vi "Start.vi"(8 "error in (no error)":errorcluster, 11 "MQTT_Base in":refnum<class "MQTT_Base.lvclass">) -> (0 "error out":errorcluster, 1 "timed out?":bool, 3 "MQTT_Base out":refnum<class "MQTT_Base.lvclass">)   [LabVIEW 2013, in "MQTT Base.lvlib" / "MQTT_Base.lvclass"]
uses:
  MQTT_Base.lvclass
  MQTT_Base.lvclass/MQTT_Base.ctl
  Launch Async Process.vi
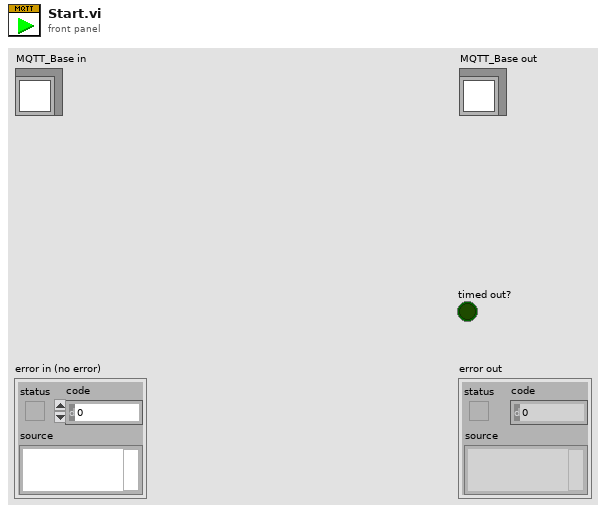
[diagram p1: front panel]
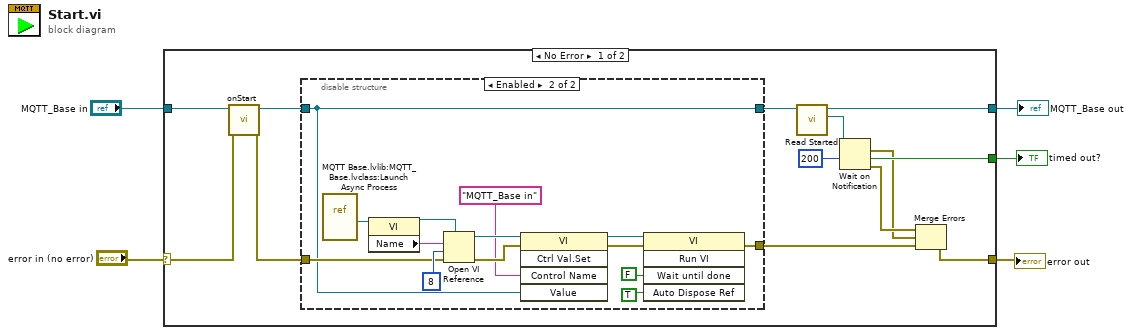
[diagram p0: block diagram]
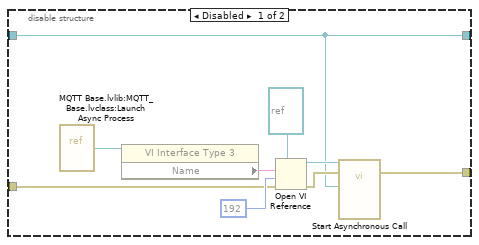
[diagram p2: hidden frame]
diagram:
  n1 = case shown="No Error" "error in (no error)" {
    selector: "error in (no error)" -> [w12 w43]
    tunnel: [w14 w43] -> w3
    tunnel: [w9 w42] -> w2
    tunnel: "MQTT_Base in" -> [w13 w42]
    tunnel: [w16 _] -> w1
    frame No Error {
      n2 = call-dynamic "onStart.vi"("error in (no error)"=w12, "MQTT_Base in"=w13) -> ("error out"=w11:errorcluster, "MQTT_Base out"=w8:refnum<class "MQTT_Base.lvclass">)  [unwired: 8 in]
      n3 = disable-structure shown="Enabled" {
        disable-tunnel: w11 -> [w23 w37]
        disable-tunnel: w8 -> [w21 w28]
        disable-tunnel: [w22 w32] -> w7
        disable-tunnel: [w21 w28] -> w6
        frame Disabled {
          n4 = vi-ref "MQTT Base.lvlib:MQTT_Base.lvclass:Launch Async Process.vi"() -> (w19:refnum<vi>)
          n5 = property class="VI Interface Type 3"(reference=w19) -> ("Name"=w27:string)  [unwired: 1 in, 2 out]
          n6 = Open VI Reference(type specifier VI Refnum (for type only)=refnum<vi> refnum ("reference out"), vi path=w27, options=192, error in (no error)=w23) -> (vi reference=w26:refnum<vi>, error out=w25:errorcluster)  [unwired: 2 in]
          n7 = call-by-ref "Start Asynchronous Call"(reference=w26, error in=w25, "MQTT_Base in"=w21) -> (error out=w22:errorcluster)  [unwired: 11 in, 1 out]
        }
        frame Enabled {
          n8 = vi-ref "MQTT Base.lvlib:MQTT_Base.lvclass:Launch Async Process.vi"() -> (w41:refnum<vi>)
          n9 = property class="VI"(reference=w41) -> (reference out=w39:refnum<vi>, "Name"=w40:string)  [unwired: 1 in, 1 out]
          n10 = Open VI Reference(type specifier VI Refnum (for type only)=w39, vi path=w40, options=8, error in (no error)=w37) -> (vi reference=w30:refnum<vi>, error out=w31:errorcluster)  [unwired: 2 in]
          n11 = invoke class="VI" method="Ctrl Val.Set"(reference=w30, error in=w31, "Control Name"="MQTT_Base in", "Value"=w28) -> (reference out=w35:refnum<vi>, error out=w36:errorcluster)  [unwired: 1 in, 3 out]
          n12 = invoke class="VI" method="Run VI"(reference=w35, error in=w36, "Wait until done"=FALSE ("Wait Until Done"), "Auto Dispose Ref"=TRUE ("Auto Dispose Reference")) -> (error out=w32:errorcluster)  [unwired: 1 in, 4 out]
        }
      }
      n13 = call "Read Started.vi"("MQTT_Base in"=w6) -> ("Started"=w15:refnum<notifier>, "MQTT_Base out"=w9:refnum<class "MQTT_Base.lvclass">)  [unwired: 8 in, 1 out]
      n14 = Wait on Notification(notifier=w15, timeout in ms (-1)=200) -> (notification=w10:errorcluster, timed out?=w16:bool, error out=w17:errorcluster)  [unwired: 2 in, 1 out]
      n15 = Merge Errors(w17, w10, w7) -> (w14:errorcluster)
    }
    frame Error {
    }
  }
  "error out" <- w3
  "MQTT_Base out" <- w2
  "timed out?" <- w1
